vi "add.vi"(5 "y":dbl, 6 "x":dbl) -> (4 "z":dbl)   [LabVIEW 2019]
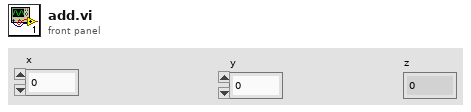
[diagram p1: front panel]
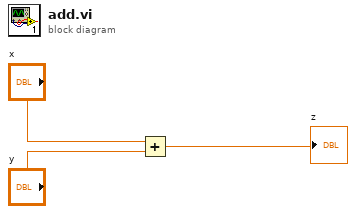
[diagram p0: block diagram]
diagram:
  n1 = Add(x="x", y="y") -> (x+y=→"z":dbl)
